vi "XRS450 SPI Gyro.vi"() -> ()   [LabVIEW 2025]
doc: "XRS450 SPI Gyro Example\n\nThis example shows how to use the Analog Devices XRS450 gyro connected to the SPI port on the RoboRIO.\n\nThis example expects a USB cable connected from your development PC to the Type B USB Jack (next to the power input) on the roboRIO.\n\nThis example expects the Driver Station to be running."
uses:
  <vilib>/Rock Robotics/SystemInterfaces/spilib/spi_bus.ctl
  <vilib>/Rock Robotics/WPI/Gyro/WPI_GyroXRS450_SPI_Open.vi
panel:
  out "Calibrated?":bool
  in  "Reset Angle?":bool
  out "Device Found":bool
  in  "stop":bool
  out "Angle":dbl(knob) scale=0.0..360.0
  in  "SPI Bus":T1
  in  "Sample Rate (Hz)":dbl=1000.0 min=50.0 max=20000.0 format="%#_13g"
  # "Set these inputs before running."
  # "This can be set while running."
  # "This will display the current gyro angle."
  # "This shows wiring for the Analog Devices XRS450 gyro.  It can be plugged directly into the SPI port."
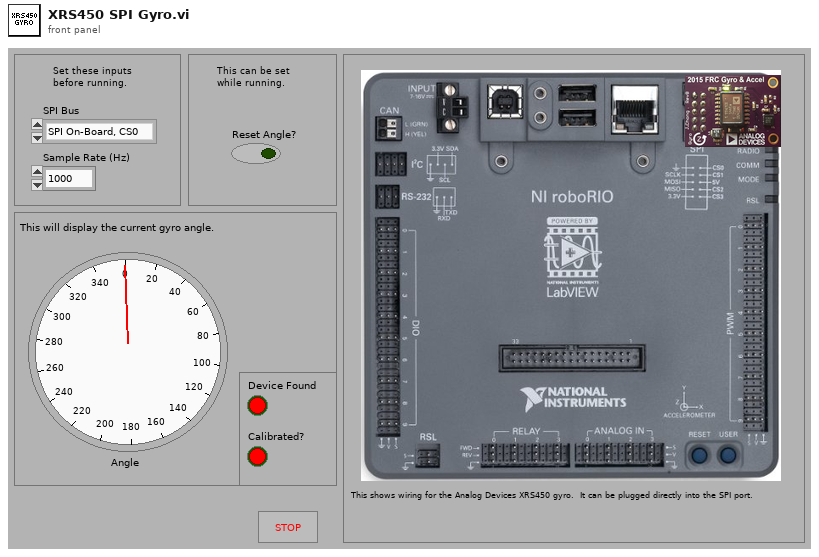
[diagram p1: front panel]
types:
  T1 = typedef "spi_bus.ctl" = enum16{"SPI On-Board, CS0", "SPI On-Board, CS1", "SPI On-Board, CS2", "SPI On-Board, CS3", "SPI MXP", "Invalid"}
  T2 = typedef "WPI_GyroDevRef.ctl" = cluster{"DevStatus":errorcluster, "Analog Channel":T3, "Gain (VoltsPerDegree/Second)":dbl, "Gyro Type":enum16{"Analog", "XRS450"}, "Handle":i32, "SPI Bus":T1, "Device Found":bool, "Sample Rate":dbl, "Calibrate On Open":bool, "Offset":dbl}
  T3 = typedef "FPGA_AIChannel.ctl" = enum8{"AI 0", "AI 1", "AI 2", "AI 3", "AI MXP 0", "AI MXP 1", "AI MXP 2", "AI MXP 3", "Invalid"}
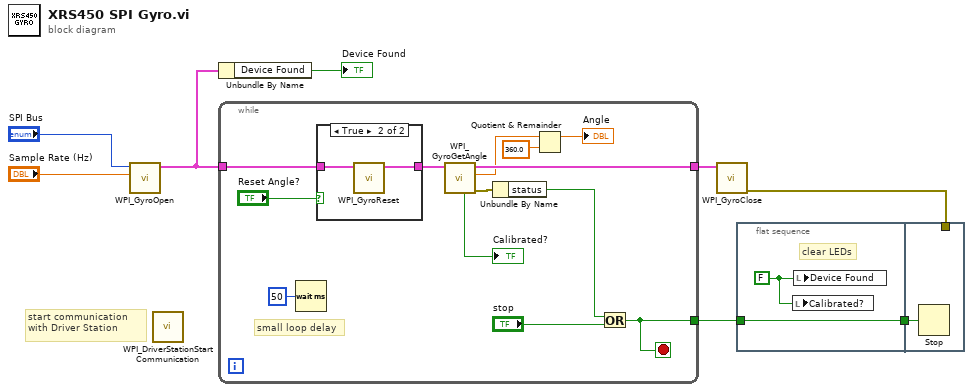
[diagram p0: block diagram]
diagram:
  # "start communication with Driver Station"
  n1 = call-poly <vilib>:"WPI_GyroOpen.vi"("Sample Rate (Hz)"="Sample Rate (Hz)", "SPI Bus"="SPI Bus") -> ("GyroDevRef"=w4:T2)  [unwired: 7 in, 2 out]
  n2 = call <vilib>:"WPI_DriverStationStart Communication.vi"() -> ()  [unwired: 12 in]
  n3 = Unbundle By Name(w4) -> ("Device Found"=→"Device Found":bool)
  n4 = while {
    tunnel: w4 -> [w17]
    tunnel: [w14] -> w6
    tunnel: [w12] -> w7
    stop <- w14 stop-if-true
    # "small loop delay"
    n5 = Wait (ms)(milliseconds to wait=u32 50) -> ()  [unwired: 1 out]
    n6 = case shown="True" "Reset Angle?" {
      tunnel: w17 -> [w22 w24]
      tunnel: [w22 w23] -> w13
      frame False {
      }
      frame True {
        n7 = call <vilib>:"WPI_GyroReset.vi"("GyroDevRef"=w24) -> ("GyroDevRef"=w23:T2)  [unwired: 9 in, 1 out]
      }
    }
    n8 = call <vilib>:"WPI_GyroGetAngle.vi"("GyroDevRef"=w13) -> ("error out"=w10:errorcluster, "Angle"=w11:dbl, "GyroDevRef"=w12:T2, "Calibrated?"=→"Calibrated?":bool)  [unwired: 6 in, 1 out]
    n9 = Unbundle By Name(w10) -> ("status"=w15:bool)
    n10 = Quotient & Remainder(x=w11, y=360.0) -> (x-y*floor(x/y)=→"Angle":dbl)  [unwired: 1 out]
    n11 = Or(x=w15, y="stop") -> (x .or. y?=w14:bool)
  }
  n12 = call <vilib>:"WPI_GyroClose.vi"("GyroDevRef"=w7) -> ("error out"=w5:errorcluster)  [unwired: 10 in]
  n13 = flat-sequence {
    tunnel: w6 -> [w26]
    tunnel: [w26] -> w1
    tunnel: w5 -> [_]
    tunnel: w1 -> [w27]
    frame #0 {
      w25 = FALSE ("Device Found")
      # "clear LEDs"
      n14 = local write "Calibrated?"(w25) -> ()
      n15 = local write "Device Found"(w25) -> ()
    }
    frame #1 {
      n16 = Stop(stop? (T)=w27) -> ()
    }
  }
